vi "Write Session.TCPIP.KeepAliveInterval.vi"(8 "error in (no error)":errorcluster, 10 "Session.TCPIP.KeepAliveInterval":dbl, 11 "SLSC Interface in":refnum<class "SLSC Interface.lvclass">) -> (0 "error out":errorcluster, 3 "SLSC Interface out":refnum<class "SLSC Interface.lvclass">)   [LabVIEW 2015, in "SLSC Interface.lvclass"]
uses:
  SLSC Interface.lvclass
  SLSC Interface.lvclass/SLSC Interface.ctl
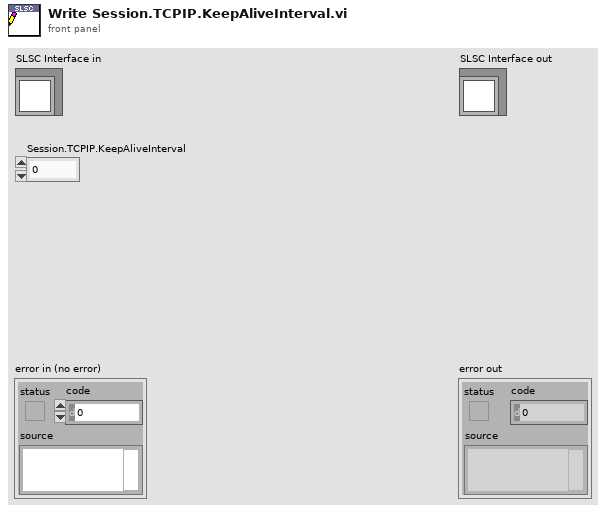
[diagram p1: front panel]
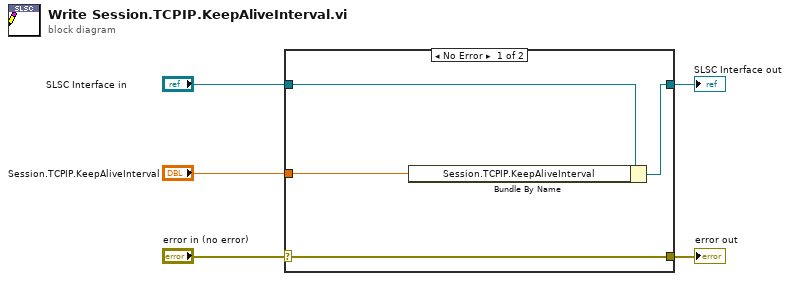
[diagram p0: block diagram]
diagram:
  n1 = case shown="No Error" "error in (no error)" {
    selector: "error in (no error)" -> [w9 w10]
    tunnel: [w9 w10] -> w4
    tunnel: [w7 w11] -> w2
    tunnel: "SLSC Interface in" -> [w8 w11]
    tunnel: "Session.TCPIP.KeepAliveInterval" -> [w6 _]
    frame No Error {
      n2 = Bundle By Name(cluster=w8, "Session.TCPIP.KeepAliveInterval"=w6) -> (w7:refnum<class "SLSC Interface.lvclass">)
    }
    frame Error {
    }
  }
  "error out" <- w4
  "SLSC Interface out" <- w2
